vi "NXT_HINDBRAIN IR Data To String.vi"(1 "_irData":T1) -> (0 "String":string)   [LabVIEW 2012, in "Tugboat.lvrbt"]
uses:
  Tugboat.lvrbt
  irData_t.ctl
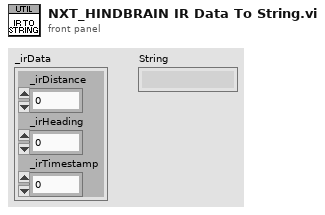
[diagram p1: front panel]
types:
  T1 = typedef "irData_t.ctl" = cluster{"_irDistance":i32, "_irHeading":i32, "_irTimestamp":u32}
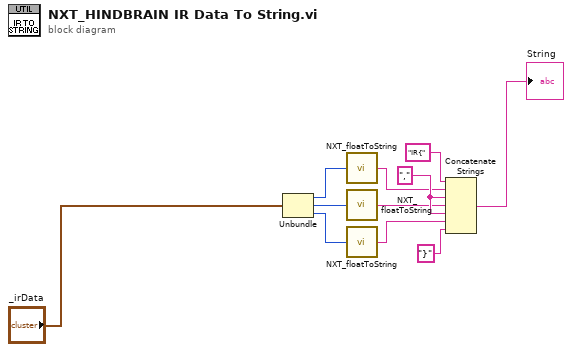
[diagram p0: block diagram]
diagram:
  w8 = "," ("string")
  n1 = Unbundle("_irData") -> ("_irDistance"=w1:i32, "_irHeading"=w2:i32, "_irTimestamp"=w3:u32)
  n2 = call <vilib>:"NXT_floatToString.vi"("number"=w1) -> ("string"=w5:string)
  n3 = call <vilib>:"NXT_floatToString.vi"("number"=w2) -> ("string"=w6:string)
  n4 = call <vilib>:"NXT_floatToString.vi"("number"=w3) -> ("string"=w7:string)
  n5 = Concatenate Strings("IR{" ("string"), w5, w8, w6, w8, w7, "}" ("string")) -> (→"String":string)
